vi "FMtsl257TekVI.vi"() -> ()   [LabVIEW 2017]
uses:
  <instrlib>/Tektronix 7000 Series/Public/Data/Read (Single Waveform).vi
  <instrlib>/Tektronix 7000 Series/Tektronix 7000 Series.lvlib
panel:
  in  "Maximum Time (10000 ms)":u32=10000
  in  "Probe Attenuation (10)":dbl=10.0
  in  "Channel (0: Channel 1)":u16(ring) format="%#_5f" items=["Channel 1", "Channel 2", "Channel 3", "Channel 4", "Math 1", "Math 2", "Math 3", "Math 4", "Reference 1", "Reference 2", "Reference 3", "Reference 4"]
  in  "VISA Resource Name":refnum<visa-resource-name>
  out "Waveform Graph 2":waveform(dbl)(graph)
  out "Waveform Graph":dynamicdata(graph)
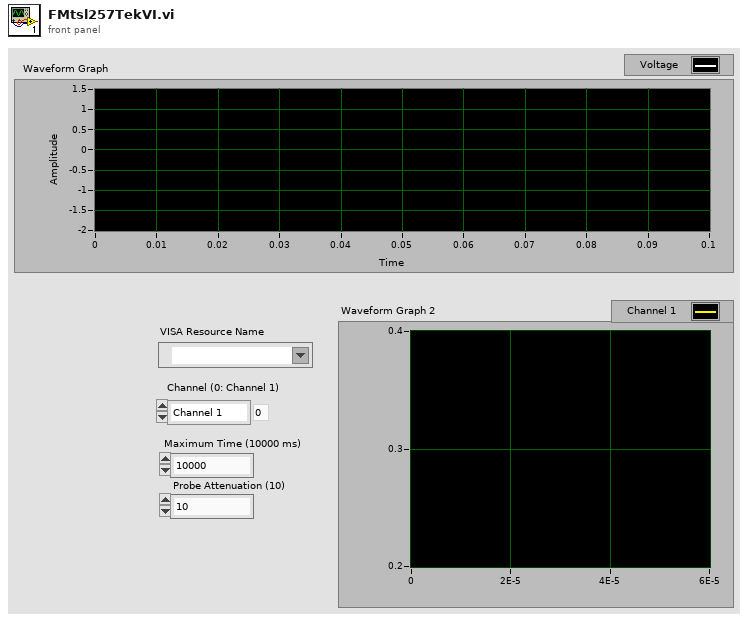
[diagram p1: front panel]
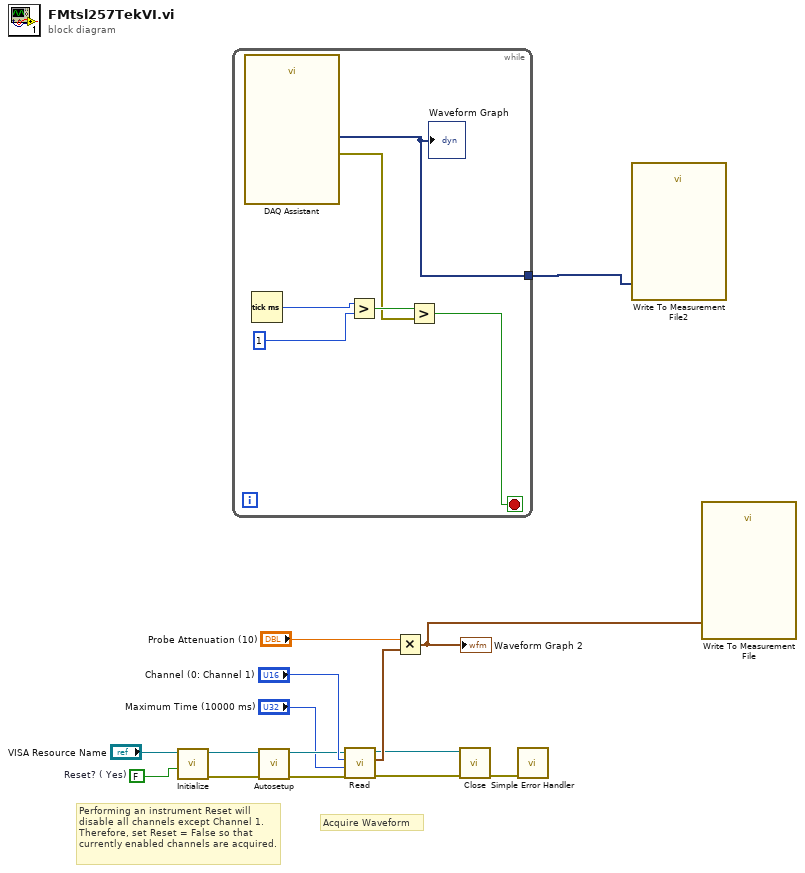
[diagram p0: block diagram]
diagram:
  w3 = FALSE  # Reset? ( Yes)
  # "Performing an instrument Reset will disable all channels except Channel 1. Therefore, set Reset = False so that currently enabled channels are acquired."
  # "Acquire Waveform"
  n1 = call <instrlib>:"Initialize.vi"("Reset? ( Yes)"=w3, "VISA resource name"="VISA Resource Name") -> ("error out"=w7:errorcluster, "VISA resource name out"=w8:refnum<visa-resource-name>)  [unwired: 8 in]
  n2 = while {
    tunnel: [w19] -> w1
    stop <- w17 stop-if-true
    n3 = call "DAQ Assistant"() -> ("data"=w19:dynamicdata, "error out"=w16:errorcluster)  [unwired: 17 in, 1 out]
    "Waveform Graph" <- w19
    n4 = Tick Count (ms)() -> (millisecond timer value=w20:u32)
    n5 = Greater?(x=w20, y=1) -> (0:w18:bool)
    n6 = Greater?(x=w18, y=w16) -> (0:w17:bool)
  }
  n7 = call <instrlib>:"Autosetup.vi"("error in (no error)"=w7, "VISA resource name"=w8) -> ("error out"=w5:errorcluster, "VISA resource name out"=w6:refnum<visa-resource-name>)  [unwired: 8 in]
  n8 = call-poly <instrlib>:"Read.vi"("error in (no error)"=w5, "Maximum Time (10000 ms)"="Maximum Time (10000 ms)", "Channel (0: Channel 1)"="Channel (0: Channel 1)", "VISA resource name"=w6) -> ("error out"=w10:errorcluster, "Waveform Data"=w12:waveform(dbl), "VISA resource name out"=w11:refnum<visa-resource-name>)  [unwired: 5 in]
  n9 = Multiply(x="Probe Attenuation (10)", y=w12) -> (x*y=w2:waveform(dbl))
  "Waveform Graph 2" <- w2
  n10 = call <instrlib>:"Close.vi"("error in (no error)"=w10, "VISA resource name"=w11) -> ("error out"=w15:errorcluster)  [unwired: 9 in]
  n11 = call <vilib>:"Simple Error Handler.vi"("error in (no error)"=w15) -> ()  [unwired: 4 in, 5 out]
  n12 = call "Write To Measurement File2"("Signals"=w1) -> ()  [unwired: 16 in, 3 out]
  n13 = call "Write To Measurement File"("Signals"=w2) -> ()  [unwired: 16 in, 3 out]
